vi "thcd_get_ahy.vi"(6 "err_in":errorcluster, 7 "thcd_visa":refnum<visa-resource-name>, 9 "thcd_ch":T1=enum."1", 10 "thcd_b2r":u32, 11 "thcd_delay":u32=500) -> (0 "thcd_st":bool, 1 "thcd_res_msg":string, 2 "thcd_res_str":string, 3 "thcd_res":i32, 4 "err_out":errorcluster, 5 "thcd_visa":refnum<visa-resource-name>)   [LabVIEW 2019]
uses:
  thcd_controls/ctrl_chn_thcd.ctl
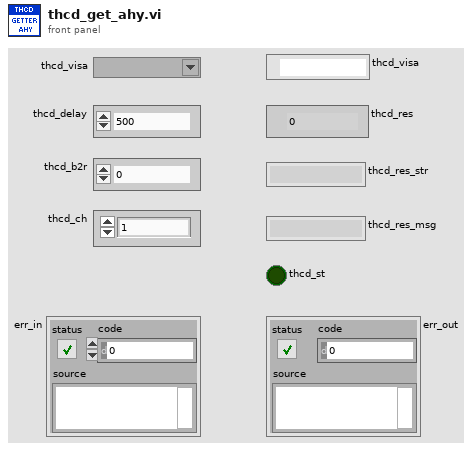
[diagram p1: front panel]
types:
  T1 = typedef "ctrl_chn_thcd.ctl" = enum8{"ERR", "1", "2", "3", "4"}
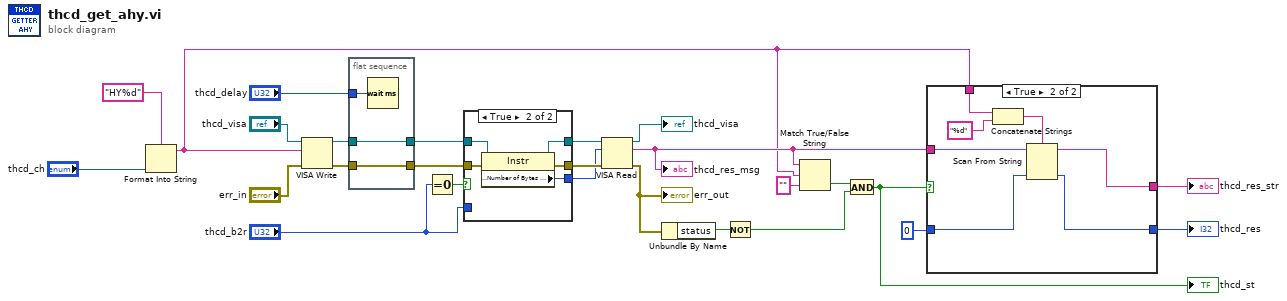
[diagram p0: block diagram]
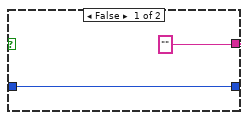
[diagram p3: hidden frame]
diagram:
  n1 = Format Into String(format string="HY%d", "thcd_ch") -> (resulting string=w8:string)  [unwired: 2 in, 1 out]
  n2 = VISA Write(VISA resource name="thcd_visa", write buffer=w8, error in (no error)="err_in") -> (VISA resource name out=w24:refnum<visa-resource-name>, error out=w26:errorcluster)  [unwired: 1 out]
  n3 = flat-sequence {
    tunnel: w26 -> [w28]
    tunnel: [w28] -> w25
    tunnel: w24 -> [w27]
    tunnel: [w27] -> w23
    tunnel: "thcd_delay" -> [w29]
    frame #0 {
      n4 = Wait (ms)(milliseconds to wait=w29) -> ()  [unwired: 1 out]
    }
  }
  n5 = Equal To 0?(x="thcd_b2r") -> (x = 0?=w5:bool)
  n6 = case shown="True" w5 {
    tunnel: w25 -> [w31 w37]
    tunnel: w23 -> [w32 w36]
    tunnel: [w32 w35] -> w22
    tunnel: [w31 w34] -> w21
    tunnel: [w30 w33] -> w4
    tunnel: "thcd_b2r" -> [w30 _]
    frame False {
    }
    frame True {
      n7 = property class="Instr"(reference=w36, error in=w37) -> (reference out=w35:refnum<visa-resource-name>, error out=w34:errorcluster, "Serial Settings:Number of Bytes at Serial Port"=w33:u32)
    }
  }
  n8 = VISA Read(VISA resource name=w22, byte count=w4, error in (no error)=w21) -> (VISA resource name out=→"thcd_visa":refnum<visa-resource-name>, read buffer=w14:string, error out=w15:errorcluster)  [unwired: 1 out]
  "err_out" <- w15
  "thcd_res_msg" <- w14
  n9 = Unbundle By Name(w15) -> ("status"=w12:bool)
  n10 = Not(x=w12) -> (.not. x?=w10:bool)
  n11 = Match True/False String(2:"" ("false string"), 3:w8, 4:w14) -> (0:w11:bool)  [unwired: 1 out]
  n12 = And(x=w11, y=w10) -> (x .and. y?=w9:bool)
  "thcd_st" <- w9
  n13 = case shown="True" w9 {
    tunnel: w14 -> [_ w44]
    tunnel: w8 -> [_ w43]
    tunnel: [w38 w42] -> w7
    tunnel: ["" w41] -> w6
    tunnel: 0 -> [w38 w40]
    frame False {
    }
    frame True {
      n14 = Concatenate Strings(w43, "%d" ("string")) -> (w45:string)
      n15 = Scan From String(format string=w45, input string=w44, default 1=w40) -> (remaining string=w41:string, output 1=w42:i32)  [unwired: 2 in, 2 out]
    }
  }
  "thcd_res_str" <- w6
  "thcd_res" <- w7
